vi "WillHeadingHitObstacle.vi"(7 "Safety offset around edges (m)":dbl=5.0, 8 "error in (no error)":errorcluster, 9 "Heading":dbl, 10 "Boat":T1 {"North" format="%#_10f"; "East" format="%#_8f"}, 11 "Obstacle.lvclass":refnum<class "Obstacle.lvclass">) -> (0 "error out":errorcluster, 3 "Any intersecting obstacles?":bool)   [LabVIEW 2013, in "Obstacle.lvclass"]
doc: "This VI looks through each segment of the given obstacle and checks whether it will collide with the segment. A safety offset around the edges is an optional input, default safety offset is given in the VI.\n\nEric Schneider, August 2014"
uses:
  Obstacle.lvclass
  Data/TypeDefs/UTM Location.ctl
  Obstacle.lvclass/Obstacle.ctl
panel:
  out "Intersecting obstacles array":bool[](array[boolean])
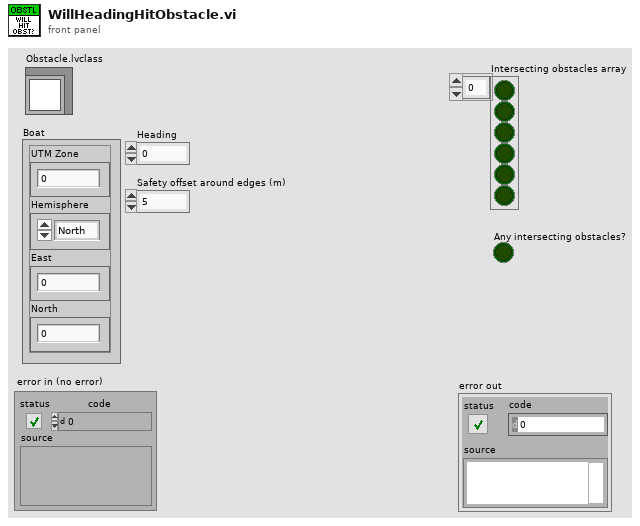
[diagram p1: front panel]
types:
  T1 = typedef "UTM Location.ctl" = cluster{"UTM Zone":dbl, "Hemisphere":enum16{"North", "South"}, "East":dbl, "North":dbl}
  T2 = cluster{"UTM Obstacle Point 2":T1, "UTM Obstacle Point 1":T1}[]
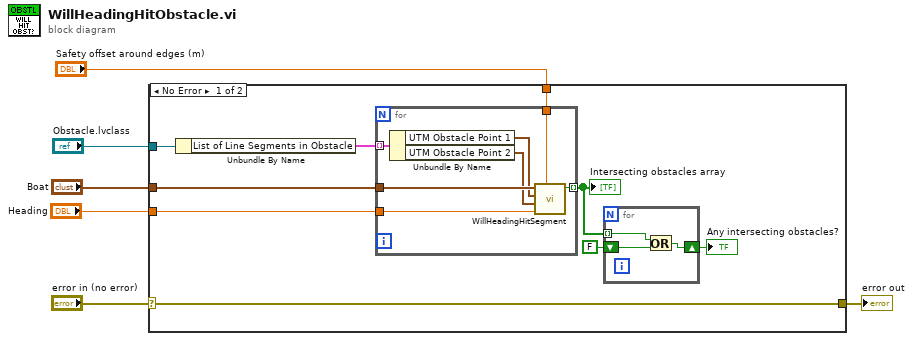
[diagram p0: block diagram]
diagram:
  n1 = case shown="No Error" "error in (no error)" {
    selector: "error in (no error)" -> [w7 w26]
    tunnel: "Obstacle.lvclass" -> [w15 _]
    tunnel: "Boat" -> [w13 _]
    tunnel: "Heading" -> [w12 _]
    tunnel: "Safety offset around edges (m)" -> [w11 _]
    tunnel: [w7 w26] -> w1
    frame No Error {
      n2 = Unbundle By Name(w15) -> ("List of Line Segments in Obstacle"=w14:T2)
      n3 = for {
        tunnel: w14 -> [w25] mode=indexing
        tunnel: w13 -> [w24]
        tunnel: w12 -> [w23]
        tunnel: w11 -> [w20]
        tunnel: [w19] -> w10 mode=indexing
        n4 = Unbundle By Name(w25) -> ("UTM Obstacle Point 1"=w22:T1, "UTM Obstacle Point 2"=w21:T1)
        n5 = call "WillHeadingHitSegment.vi"("Safety offset around edges (m)"=w20, "Heading (deg)"=w23, "Segment Point 2"=w21, "Segment Point 1"=w22, "Boat Point"=w24) -> ("Will collide"=w19:bool)  [unwired: 6 in]
      }
      "Intersecting obstacles array" <- w10
      n6 = for {
        tunnel: w10 -> [w17] mode=indexing
        shift-right: [w16] -> w8
        shift-left: FALSE -> [w18]
        n7 = Or(x=w17, y=w18) -> (x .or. y?=w16:bool)
      }
      "Any intersecting obstacles?" <- w8
    }
    frame Error {
    }
  }
  "error out" <- w1
